vi "Configure Event Timing Capture Dialog.vi"(5 "Window reference angle":dbl, 7 "capture to be edited":i32, 8 "error in (no error)":errorcluster, 10 "captures in":T2[](array[typedef]), 11 "Item Ref in":T3 format="%.0x") -> (0 "error out":errorcluster, 2 "captures out":T2[](array[typedef]), 3 "Item Ref out":T3 format="%.0x")   [LabVIEW 2013, in "Engine Simulation Toolkit System Explorer.lvlib"]
uses:
  Engine Simulation Toolkit System Explorer.lvlib
  Event Timing Capture.ctl
  Event Reference Angle Selection.ctl
  <vilib>/NI Veristand/Custom Device API/Custom Device Item Ref.ctl
  <vilib>/NI Veristand/Custom Device API/Custom Device API.lvlib
panel:
  in  "Reference angle defined":T1
  in  "Reference angle":dbl
  in  "Default end angle":dbl=1.0
  in  "Default start angle":dbl
  in  "Cancel":bool
  in  "OK":bool
  in  "Name":string
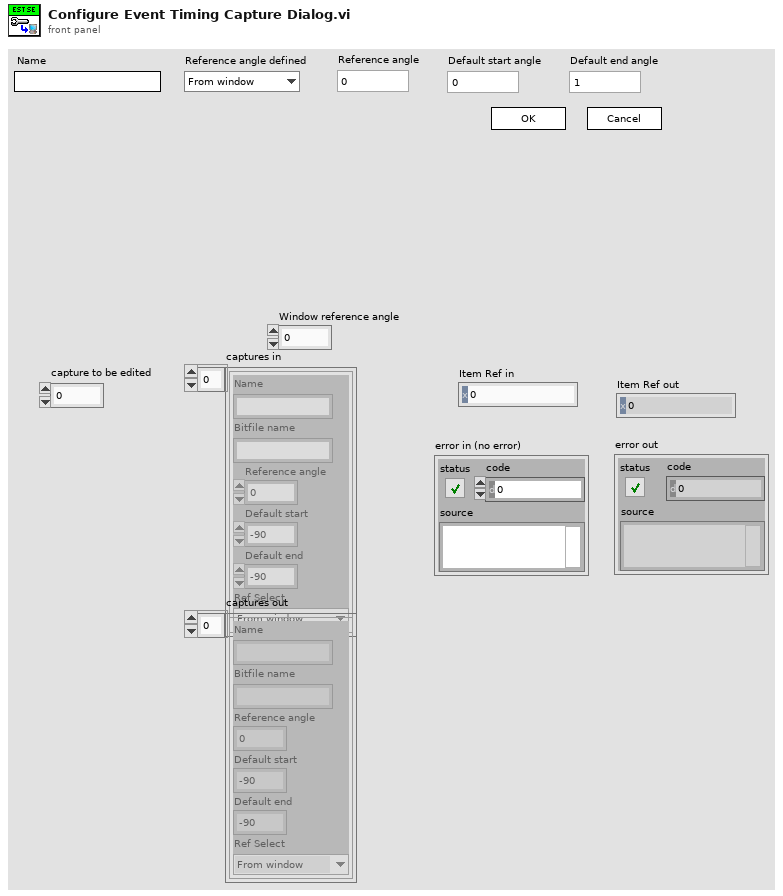
[diagram p1: front panel]
types:
  T1 = typedef "Engine Simulation Toolkit System Explorer.lvlib/Event Reference Angle Selection.ctl" = enum16{"From window", "Custom"}
  T2 = typedef "Engine Simulation Toolkit System Explorer.lvlib/Event Timing Capture.ctl" = cluster{"Name":string, "Bitfile name":string, "Reference angle":dbl, "Default start":dbl, "Default end":dbl, "Ref Select":T1}
  T3 = typedef "Custom Device API.lvlib/Custom Device Item Ref.ctl" = u64
  T4 = enum8{"Enabled", "Disabled", "Disabled and Grayed Out"}
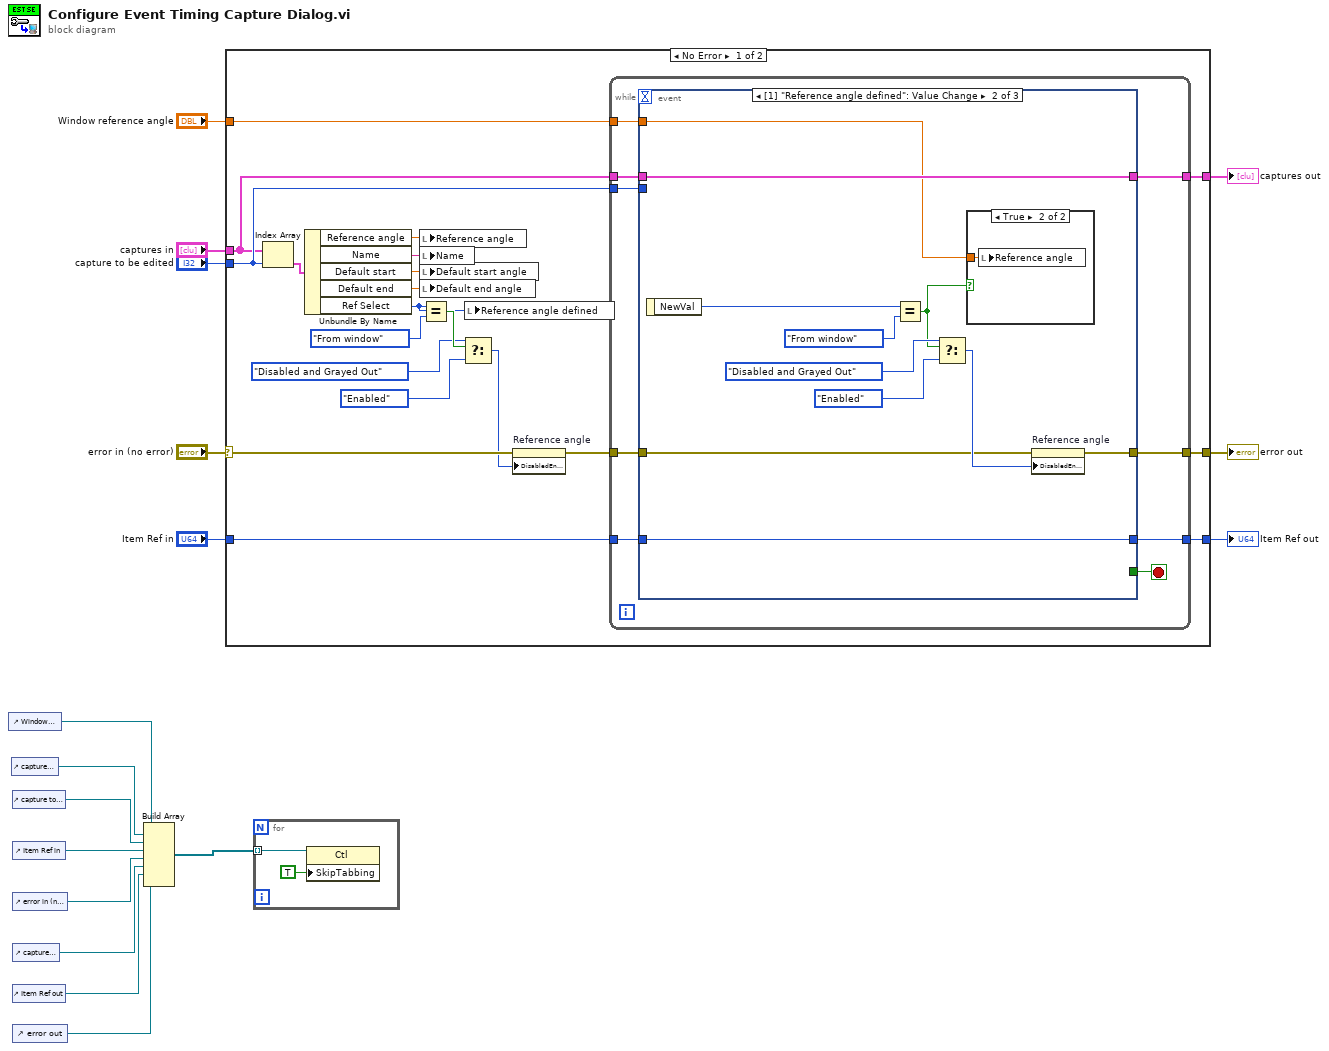
[diagram p0: block diagram]
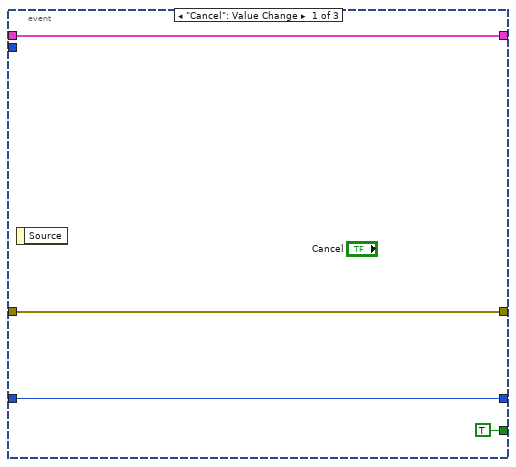
[diagram p2: hidden frame]
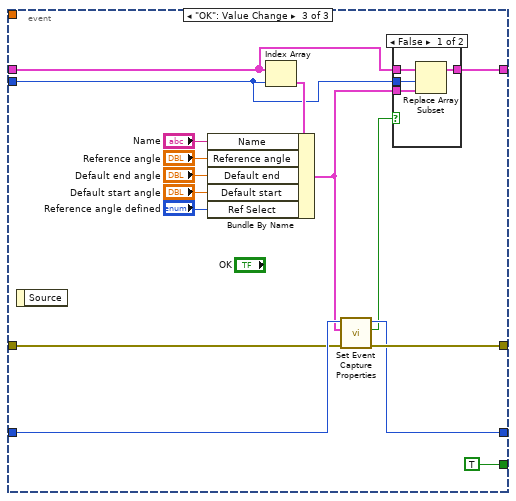
[diagram p4: hidden frame]
diagram:
  n1 = control-ref of="Window reference angle"() -> (w2:refnum<vi>)
  n2 = control-ref of="captures out"() -> (w5:refnum<vi>)
  n3 = control-ref of="capture to be edited"() -> (w11:refnum<vi>)
  n4 = control-ref of="Item Ref in"() -> (w10:refnum<vi>)
  n5 = control-ref of="error in (no error)"() -> (w9:refnum<vi>)
  n6 = control-ref of="captures in"() -> (w8:refnum<vi>)
  n7 = control-ref of="Item Ref out"() -> (w4:refnum<vi>)
  n8 = control-ref of="error out"() -> (w3:refnum<vi>)
  n9 = Build Array(w2, w5, w11, w10, w9, w8, w4, w3) -> (w7:refnum<vi>[])
  n10 = case shown="No Error" "error in (no error)" {
    selector: "error in (no error)" -> [w29 w86]
    tunnel: "captures in" -> [w35 w85]
    tunnel: "capture to be edited" -> [w36 _]
    tunnel: [w37 w86] -> w14
    tunnel: [w34 w85] -> w6
    tunnel: "Item Ref in" -> [w33 w84]
    tunnel: [w32 w84] -> w12
    tunnel: "Window reference angle" -> [w21 _]
    frame No Error {
      n11 = Index Array(array=w35, index=w36) -> (element=w30:T2)
      n12 = Unbundle By Name(w30) -> ("Reference angle"=w20:dbl, "Name"=w31:string, "Default start"=w28:dbl, "Default end"=w19:dbl, "Ref Select"=w18:T1)
      n13 = local write "Reference angle"(w20) -> ()
      n14 = local write "Name"(w31) -> ()
      n15 = local write "Default start angle"(w28) -> ()
      n16 = local write "Default end angle"(w19) -> ()
      n17 = Equal?(x=w18, y=Event_Reference_Angle_Selection."From window") -> (x = y?=w25:bool)
      n18 = Select(t=T4."Disabled and Grayed Out" ("Disabled"), s=w25, f=T4."Enabled" ("Disabled")) -> (s? t:f=w22:T4)
      n19 = local write "Reference angle defined"(w18) -> ()
      n20 = property on="Reference angle" class="DigNum (strict)"(error in=w29, "DisabledEnum"=w22) -> (error out=w27:errorcluster)  [unwired: 1 in, 1 out]
      n21 = while {
        tunnel: [w39] -> w37
        tunnel: w27 -> [w46]
        tunnel: w36 -> [w45]
        tunnel: w33 -> [w42]
        tunnel: [w41] -> w32
        tunnel: w21 -> [w38]
        tunnel: w35 -> [w44]
        tunnel: [w43] -> w34
        stop <- w40 stop-if-true
        n22 = event shown="[1] \"Reference angle defined\": Value Change" {
          selector: _ -> [_ _ _]
          dyn-events: _ -> [_ _ _]
          timeout: _ -> [_ _ _]
          tunnel: [w50 w54 w73] -> w39
          tunnel: w46 -> [w50 w55 w69]
          tunnel: w45 -> [_ _ w75]
          tunnel: w44 -> [w49 w61 w76]
          tunnel: [w49 w61 w74] -> w43
          tunnel: w42 -> [w48 w60 w72]
          tunnel: [w48 w60 w71] -> w41
          tunnel: [TRUE _ TRUE] -> w40
          tunnel: w38 -> [_ w51 _]
          event "Cancel": Value Change {
            n23 = event-data() -> ()  [unwired: 1 in, 1 out]
          }
          event Value Change {
            n24 = event-data() -> ("NewVal"=w53:T1)  [unwired: 1 in]
            n25 = Equal?(x=w53, y=Event_Reference_Angle_Selection."From window") -> (x = y?=w52:bool)
            n26 = Select(t=T4."Disabled and Grayed Out" ("Disabled"), s=w52, f=T4."Enabled" ("Disabled")) -> (s? t:f=w59:T4)
            n27 = case shown="True" w52 {
              tunnel: w51 -> [_ w62]
              frame False {
              }
              frame True {
                n28 = local write "Reference angle"(w62) -> ()
              }
            }
            n29 = property on="Reference angle" class="DigNum (strict)"(error in=w55, "DisabledEnum"=w59) -> (error out=w54:errorcluster)  [unwired: 1 in, 1 out]
          }
          event "OK": Value Change {
            n30 = event-data() -> ()  [unwired: 1 in, 1 out]
            n31 = Index Array(array=w76, index=w75) -> (element=w77:T2)
            n32 = Bundle By Name(cluster=w77, "Name"="Name", "Reference angle"="Reference angle", "Default end"="Default end angle", "Default start"="Default start angle", "Ref Select"="Reference angle defined") -> (w64:T2)
            n33 = call "Set Event Capture Properties.vi"("error in (no error)"=w69, "capture"=w64, "Item Ref in"=w72) -> ("error out"=w73:errorcluster, "failed"=w70:bool, "Item Ref out"=w71:T3)  [unwired: 6 in]
            n34 = case shown="False" w70 {
              tunnel: w76 -> [w82 w83]
              tunnel: w75 -> [w81 _]
              tunnel: [w80 w83] -> w74
              tunnel: w64 -> [w79 _]
              frame False {
                n35 = Replace Array Subset(array=w82, new element=w79, index=w81) -> (w80:T2[])
              }
              frame True {
              }
            }
          }
        }
      }
    }
    frame Error {
    }
  }
  "error out" <- w14
  "Item Ref out" <- w12
  "captures out" <- w6
  n36 = for {
    tunnel: w7 -> [w88] mode=indexing
    n37 = property class="Ctl"(reference=w88, "SkipTabbing"=TRUE ("Skip When Tabbing")) -> ()  [unwired: 1 in, 2 out]
  }
